vi "PacketLostAscan(SubVI).vi"(8 "Enable log":bool, 10 "Status":T1={"CRC8Good"=TRUE, "PackEndGood"=TRUE, "MWFind"=TRUE, "PackToSmall"=FALSE, "offset"=4}, 11 "UNDT_Cl1":T2 {"Gain Coeff" format="%#_6e"; "Reserve 1" format="%02x"; "Mux TX/RX" format="%02x"; "ScanDelay" format="%02x"; "PacketCounter" format="%08x"; "SamplingInterval" format="%#_6e"; "Lose Packet" format="%08x"; "EncodersParam2" format="%016x"; "EncodersParam1" format="%016x"; "CRC 8" format="%02x"; "N chanel" format="%02x"; "N tick" format="%02x"; "Ncycle" format="%04x"; "FrameFormatVersion" format="%02x"; "MagicWord" format="%.0x"}) -> (0 "Cluster":cluster{"CRC8_bad":u32, "PackEnd_bad":u32}, 1 "Lost":bool, 3 "CountLostPack out":u32, 4 "Stat":u64[][](array[numeric]))   [LabVIEW 2017]
uses:
  Control_EU/UNDT_ClusterPackRevers (Type).ctl
  Control_EU/Status_pack5.ctl
panel:
  out "Array":string[](array[string])
  out "PacketNumberLast":u32
  # "PacketCounter--N chanel--GlobalTime2--GlobalTime1--N tick--Ncycle--Gain--PacketCounter"
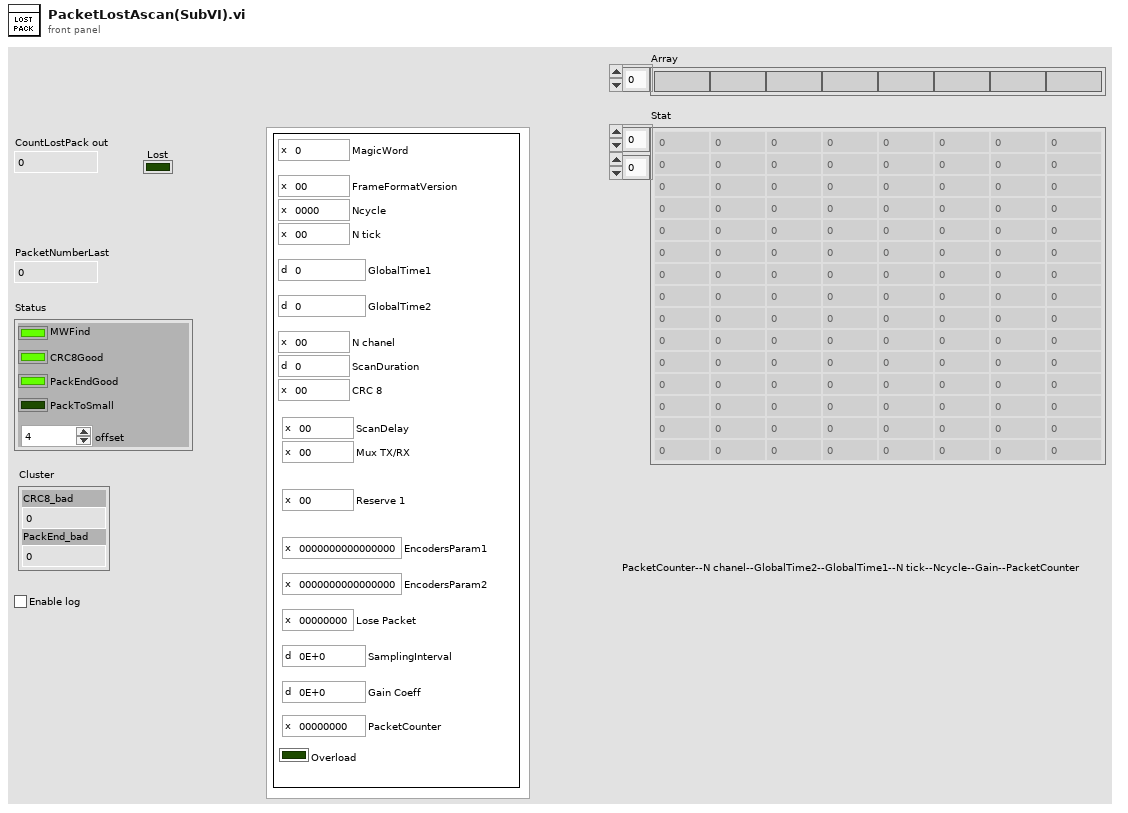
[diagram p1: front panel]
types:
  T1 = typedef "Status_pack5.ctl" = cluster{"CRC8Good":bool, "PackEndGood":bool, "MWFind":bool, "PackToSmall":bool, "offset":i32}
  T2 = typedef "UNDT_ClusterPackRevers (Type).ctl" = cluster{"PacketCounter":u32, "Gain Coeff":sgl, "SamplingInterval":sgl, "Lose Packet":u32, "EncodersParam2":u64, "EncodersParam1":u64, "Reserve 1":u8, "Mux TX/RX":u8, "ScanDelay":u16, "CRC 8":u8, "ScanDuration":u16, "N chanel":u8, "GlobalTime2":u32, "GlobalTime1":u32, "N tick":u8, "Ncycle":u16, "FrameFormatVersion":u8, "MagicWord":u32, "Overload":bool}
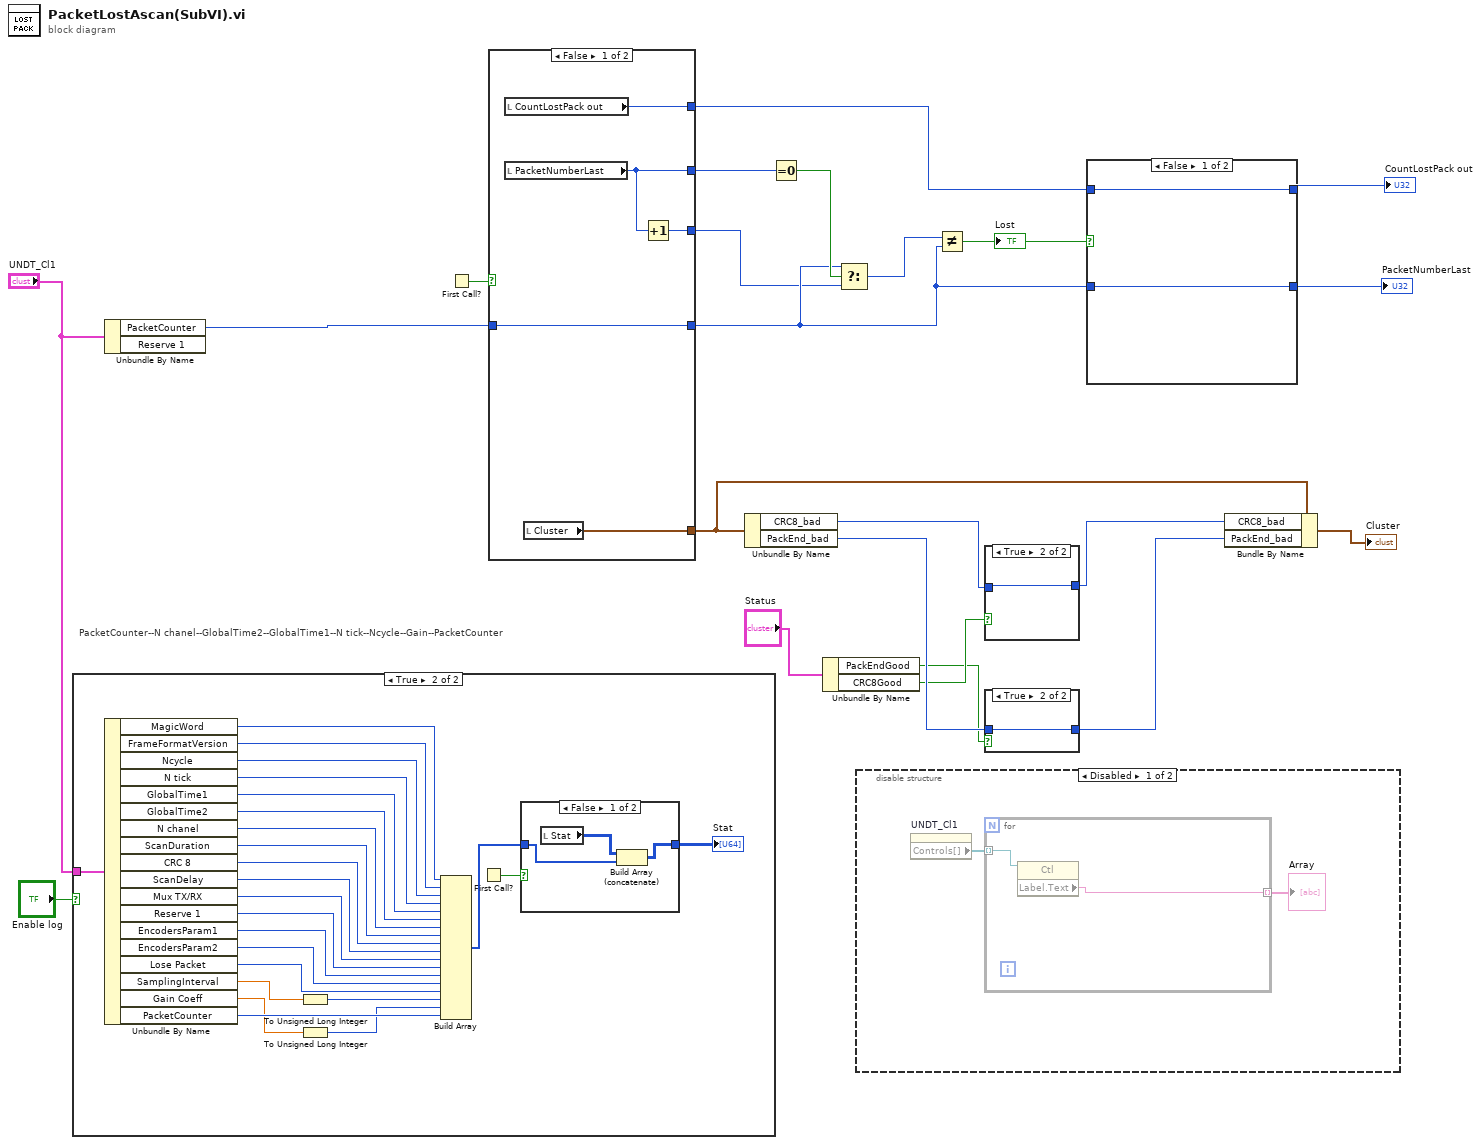
[diagram p0: block diagram]
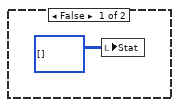
[diagram p3: hidden frame]
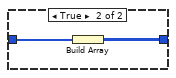
[diagram p4: hidden frame]
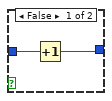
[diagram p5: hidden frame]
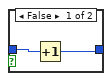
[diagram p6: hidden frame]
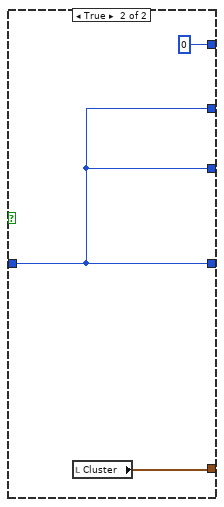
[diagram p7: hidden frame]
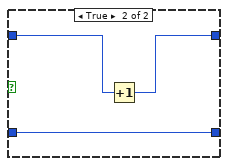
[diagram p8: hidden frame]
diagram:
  # "PacketCounter--N chanel--GlobalTime2--GlobalTime1--N tick--Ncycle--Gain--PacketCounter"
  n1 = case shown="True" "Enable log" {
    tunnel: "UNDT_Cl1" -> [_ w26]
    frame False {
      n2 = local write "Stat"(u64[][] [] ("Stat")) -> ()
    }
    frame True {
      n3 = Unbundle By Name(w26) -> ("MagicWord"=w31:u32, "FrameFormatVersion"=w47:u8, "Ncycle"=w46:u16, "N tick"=w45:u8, "GlobalTime1"=w44:u32, "GlobalTime2"=w43:u32, "N chanel"=w41:u8, "ScanDuration"=w40:u16, "CRC 8"=w39:u8, "ScanDelay"=w38:u16, "Mux TX/RX"=w37:u8, "Reserve 1"=w36:u8, "EncodersParam1"=w35:u64, "EncodersParam2"=w34:u64, "Lose Packet"=w33:u32, "SamplingInterval"=w30:sgl, "Gain Coeff"=w28:sgl, "PacketCounter"=w32:u32)
      n4 = To Unsigned Long Integer(number=w30) -> (unsigned 32bit integer=w29:u32)
      n5 = To Unsigned Long Integer(number=w28) -> (unsigned 32bit integer=w27:u32)
      n6 = Build Array(w31, w47, w46, w45, w44, w43, w41, w40, w39, w38, w37, w36, w35, w34, w33, w29, w27, w32) -> (w42:u64[])
      n7 = First Call?() -> (First Call?: T/F=w24:bool)
      n8 = case shown="False" w24 {
        tunnel: w42 -> [w49 w52]
        tunnel: [w48 w51] -> w25
        frame False {
          n9 = local read "Stat"() -> (w50:u64[][])
          n10 = Build Array (concatenate)(w50, w49) -> (w48:u64[][])
        }
        frame True {
          n11 = Build Array(w52) -> (w51:u64[][])
        }
      }
      "Stat" <- w25
    }
  }
  n12 = Unbundle By Name("UNDT_Cl1") -> ("PacketCounter"=w5:u32)  [unwired: 1 out]
  n13 = First Call?() -> (First Call?: T/F=w18:bool)
  n14 = case shown="False" w18 {
    tunnel: [w54 w59] -> w17
    tunnel: [w57 w59] -> w16
    tunnel: w5 -> [w57 w59]
    tunnel: [w56 u32 0 ("CountLostPack out")] -> w15
    tunnel: [w55 w59] -> w14
    tunnel: [w53 w58] -> w11
    frame False {
      n15 = local read "CountLostPack out"() -> (w56:u32)
      n16 = local read "PacketNumberLast"() -> (w54:u32)
      n17 = local read "Cluster"() -> (w53:cluster{"CRC8_bad":u32, "PackEnd_bad":u32})
      n18 = Increment(x=w54) -> (x+1=w55:u32)
    }
    frame True {
      n19 = local read "Cluster"() -> (w58:cluster{"CRC8_bad":u32, "PackEnd_bad":u32})
    }
  }
  n20 = Unbundle By Name(w11) -> ("CRC8_bad"=w10:u32, "PackEnd_bad"=w12:u32)
  n21 = Equal To 0?(x=w17) -> (x = 0?=w20:bool)
  n22 = Unbundle By Name("Status") -> ("PackEndGood"=w7:bool, "CRC8Good"=w8:bool)
  n23 = Select(t=w16, s=w20, f=w14) -> (s? t:f=w21:u32)
  n24 = disable-structure shown="Disabled" {
    frame Disabled {
      n25 = property on="UNDT_Cl1" class="Clust (strict)"() -> ("Controls[]"=w62:refnum<vi>[])  [unwired: 2 in, 2 out]
      n26 = for {
        tunnel: w62 -> [w64] mode=indexing
        tunnel: [w63] -> w61 mode=indexing
        n27 = property class="Ctl"(reference=w64) -> ("Label.Text"=w63:string)  [unwired: 1 in, 2 out]
      }
      "Array" <- w61
    }
    frame Enabled {
    }
  }
  n28 = Not Equal?(x=w21, y=w16) -> (x != y?=w22:bool)
  "Lost" <- w22
  n29 = case shown="True" w8 {
    tunnel: w10 -> [w66 w67]
    tunnel: [w65 w67] -> w3
    frame False {
      n30 = Increment(x=w66) -> (x+1=w65:u32)
    }
    frame True {
    }
  }
  n31 = case shown="True" w7 {
    tunnel: w12 -> [w69 w70]
    tunnel: [w68 w70] -> w2
    frame False {
      n32 = Increment(x=w69) -> (x+1=w68:u32)
    }
    frame True {
    }
  }
  n33 = case shown="False" w22 {
    tunnel: w15 -> [w72 w74]
    tunnel: [w72 w73] -> w1
    tunnel: w16 -> [w71 w75]
    tunnel: [w71 w75] -> w19
    frame False {
    }
    frame True {
      n34 = Increment(x=w74) -> (x+1=w73:u32)
    }
  }
  "CountLostPack out" <- w1
  "PacketNumberLast" <- w19
  n35 = Bundle By Name(cluster=w11, "CRC8_bad"=w3, "PackEnd_bad"=w2) -> (→"Cluster":cluster{"CRC8_bad":u32, "PackEnd_bad":u32})
